vi "Func-엑셀 데이터를 그래프로 출력.vi"() -> ()   [LabVIEW 2015] (continued)
65\t65\t71.845\n65\t65\t71.844\n65\t65\t71.842\n65\t65\t71.84\n65\t65\t71.84\n65\t65\t71.843\n65\t65\t71.838\n65\t65\t71.837\n65\t65\t71.84\n65\t65\t71.846\n65\t65\t71.843\n65\t65\t71.844\n65\t65\t71.846\n65\t65\t71.846\n65\t65\t71.843\n65\t65\t71.832\n65\t65\t71.833\n65\t65\t71.83\n65\t65\t71.829\n65\t65\t71.828\n65\t65\t71.828\n65\t65\t71.832\n65\t65\t71.828\n65\t65\t71.827\n65\t65\t71.823\n65\t65\t71.822\n65\t65\t71.817\n65\t65\t71.814\n65\t65\t71.814\n65\t65\t71.816\n65\t65\t71.817\n65\t65\t71.811\n65\t65\t71.813\n65\t65\t71.814\n65\t65\t71.812\n65\t65\t71.806\n65\t65\t71.799\n65\t65\t71.798\n65\t65\t71.798\n65\t65\t71.793\n65\t65\t71.792\n65\t65\t71.795\n65\t65\t71.796\n65\t65\t71.801\n65\t65\t71.798\n65\t65\t71.797\n65\t65\t71.8\n65\t65\t71.798\n65\t65\t71.799\n65\t65\t71.796\n65\t65\t71.8\n65\t65\t71.803\n65\t65\t71.802\n65\t65\t71.801\n65\t65\t71.797\n65\t65\t71.796\n65\t65\t71.79\n65\t65\t71.786\n65\t65\t71.783\n65\t65\t71.781\n65\t65\t71.782\n65\t65\t71.782\n65\t65\t71.781\n65\t65\t71.781\n65\t65\t71.779\n65\t65\t71.776\n65\t65\t71.777\n65\t65\t71.773\n65\t65\t71.769\n65\t65\t71.769\n65\t65\t71.767\n65\t65\t71.763\n65\t65\t71.761\n65\t65\t71.759\n65\t65\t71.761\n65\t65\t71.754\n65\t65\t71.754\n65\t65\t71.754\n65\t65\t71.751\n65\t65\t71.752\n65\t65\t71.752\n65\t65\t71.755\n65\t65\t71.754\n65\t65\t71.756\n65\t65\t71.754\n65\t65\t71.752\n65\t65\t71.75\n65\t65\t71.75\n65\t65\t71.75\n65\t65\t71.75\n65\t65\t71.749\n65\t65\t71.746\n65\t65\t71.745\n65\t65\t71.741\n65\t65\t71.738\n65\t65\t71.739\n65\t65\t71.742\n65\t65\t71.743\n65\t65\t71.741\n65\t65\t71.741\n65\t65\t71.742\n65\t65\t71.738\n65\t65\t71.738\n65\t65\t71.736\n65\t65\t71.736\n65\t65\t71.733\n65\t65\t71.731\n65\t65\t71.73\n65\t65\t71.725\n65\t65\t71.725\n65\t65\t71.723\n65\t65\t71.721\n65\t65\t71.723\n65\t65\t71.72\n65\t65\t71.72\n65\t65\t71.719\n65\t65\t71.719\n65\t65\t71.716\n65\t65\t71.714\n65\t65\t71.714\n65\t65\t71.714\n65\t65\t71.713\n65\t65\t71.713\n65\t65\t71.714\n65\t65\t71.711\n65\t65\t71.712\n65\t65\t71.711\n65\t65\t71.711\n65\t65\t71.712\n65\t65\t71.712\n65\t65\t71.715\n65\t65\t71.712\n65\t65\t71.709\n65\t65\t71.709\n65\t65\t71.702\n65\t65\t71.7\n65\t65\t71.695\n65\t65\t71.698\n65\t65\t71.698\n65\t65\t71.698\n65\t65\t71.699\n65\t65\t71.698\n65\t65\t71.696\n65\t65\t71.693\n65\t65\t71.691\n65\t65\t71.687\n65\t65\t71.687\n65\t65\t71.687\n65\t65\t71.688\n65\t65\t71.687\n65\t65\t71.689\n65\t65\t71.689\n65\t65\t71.687\n65\t65\t71.686\n65\t65\t71.682\n65\t65\t71.685\n65\t65\t71.683\n65\t65\t71.683\n65\t65\t71.682\n65\t65\t71.679\n65\t65\t71.675\n65\t65\t71.673\n65\t65\t71.669\n65\t65\t71.67\n65\t65\t71.672\n65\t65\t71.677\n65\t65\t71.68\n65\t65\t71.679\n65\t65\t71.679\n65\t65\t71.676\n65\t65\t71.671\n65\t65\t71.671\n65\t65\t71.669\n65\t65\t71.667\n65\t65\t71.666\n65\t65\t71.667\n65\t65\t71.666\n65\t65\t71.666\n65\t65\t71.664\n65\t65\t71.664\n65\t65\t71.66\n65\t65\t71.657\n65\t65\t71.657\n65\t65\t71.652\n65\t65\t71.653\n65\t65\t71.652\n65\t65\t71.656\n65\t65\t71.655\n65\t65\t71.651\n65\t65\t71.652\n65\t65\t71.65\n65\t65\t71.644\n65\t65\t71.643\n65\t65\t71.645\n65\t65\t71.645\n65\t65\t71.645\n65\t65\t71.648\n65\t65\t71.648\n65\t65\t71.645\n65\t65\t71.645\n65\t65\t71.64\n65\t65\t71.637\n65\t65\t71.632\n65\t65\t71.634\n65\t65\t71.633\n65\t65\t71.633\n65\t65\t71.636\n65\t65\t71.637\n65\t65\t71.637\n65\t65\t71.637\n65\t65\t71.637\n65\t65\t71.636\n65\t65\t71.634\n65\t65\t71.633\n65\t65\t71.633\n65\t65\t71.627\n65\t65\t71.623\n65\t65\t71.622\n65\t65\t71.621\n65\t65\t71.617\n65\t65\t71.617\n65\t65\t71.616\n65\t65\t71.618\n65\t65\t71.616\n65\t65\t71.617\n65\t65\t71.621\n65\t65\t71.62\n65\t65\t71.622\n65\t65\t71.621\n65\t65\t71.623\n65\t65\t71.62\n65\t65\t71.613\n65\t65\t71.608\n65\t65\t71.613\n65\t65\t71.613\n65\t65\t71.606\n65\t65\t71.603\n65\t65\t71.602\n65\t65\t71.604\n65\t65\t71.595\n65\t65\t71.595\n65\t65\t71.595\n65\t65\t71.598\n65\t65\t71.597\n65\t65\t71.599\n65\t65\t71.599\n65\t65\t71.595\n65\t65\t71.594\n65\t65\t71.597\n65\t65\t71.601\n65\t65\t71.597\n65\t65\t71.593\n65\t65\t71.593\n65\t65\t71.592\n65\t65\t71.588\n65\t65\t71.584\n65\t65\t71.584\n65\t65\t71.588\n65\t65\t71.586\n65\t65\t71.582\n65\t65\t71.584\n65\t65\t71.583\n65\t65\t71.582\n65\t65\t71.584\n65\t65\t71.585\n65\t65\t71.586\n65\t65\t71.586\n65\t65\t71.584\n65\t65\t71.584\n65\t65\t71.58\n65\t65\t71.58\n65\t65\t71.58\n65\t65\t71.577\n65\t65\t71.574\n65\t65\t71.575\n65\t65\t71.575\n65\t65\t71.57\n65\t65\t71.568\n65\t65\t71.57\n65\t65\t71.57\n65\t65\t71.569\n65\t65\t71.571\n65\t65\t71.572\n65\t65\t71.572\n65\t65\t71.567\n65\t65\t71.568\n65\t65\t71.567\n65\t65\t71.562\n65\t65\t71.561\n65\t65\t71.561\n65\t65\t71.564\n65\t65\t71.562\n65\t65\t71.562\n65\t65\t71.56\n65\t65\t71.557\n65\t65\t71.557\n65\t65\t71.553\n65\t65\t71.554\n65\t65\t71.549\n65\t65\t71.548\n65\t65\t71.548\n65\t65\t71.548\n65\t65\t71.551\n65\t65\t71.553\n65\t65\t71.551\n65\t65\t71.554\n65\t65\t71.556\n65\t65\t71.555\n65\t65\t71.552\n65\t65\t71.553\n65\t65\t71.556\n65\t65\t71.555\n65\t65\t71.55\n65\t65\t71.546\n65\t65\t71.542\n65\t65\t71.536\n65\t65\t71.535\n65\t65\t71.532\n65\t65\t71.533\n65\t65\t71.532\n65\t65\t71.536\n65\t65\t71.539\n65\t65\t71.536\n65\t65\t71.534\n65\t65\t71.534\n65\t65\t71.536\n65\t65\t71.534\n65\t65\t71.531\n65\t65\t71.534\n65\t65\t71.537\n65\t65\t71.536\n65\t65\t71.537\n65\t65\t71.536\n65\t65\t71.535\n65\t65\t71.531\n65\t65\t71.528\n65\t65\t71.528\n65\t65\t71.526\n65\t65\t71.528\n65\t65\t71.527\n65\t65\t71.529\n65\t65\t71.528\n65\t65\t71.528\n65\t65\t71.523\n65\t65\t71.518\n65\t65\t71.518\n65\t65\t71.519\n65\t65\t71.52\n65\t65\t71.519\n65\t65\t71.522\n65\t65\t71.527\n65\t65\t71.523\n65\t65\t71.52\n65\t65\t71.517\n65\t65\t71.517\n65\t65\t71.512\n65\t65\t71.511\n65\t65\t71.511\n65\t65\t71.508\n65\t65\t71.509\n65\t65\t71.507\n65\t65\t71.509\n65\t65\t71.507\n65\t65\t71.509\n65\t65\t71.511\n65\t65\t71.506\n65\t65\t71.507\n65\t65\t71.505\n65\t65\t71.504\n65\t65\t71.5\n65\t65\t71.5\n65\t65\t71.502\n65\t65\t71.499\n65\t65\t71.499\n65\t65\t71.495\n65\t65\t71.495\n65\t65\t71.491\n65\t65\t71.489\n65\t65\t71.491\n65\t65\t71.49\n65\t65\t71.491\n65\t65\t71.491\n65\t65\t71.492\n65\t65\t71.493\n65\t65\t71.491\n65\t65\t71.488\n65\t65\t71.492\n65\t65\t71.491\n65\t65\t71.49\n65\t65\t71.489\n65\t65\t71.486\n65\t65\t71.486\n65\t65\t71.48\n65\t65\t71.476\n65\t65\t71.476\n65\t65\t71.473\n65\t65\t71.474\n65\t65\t71.475\n65\t65\t71.477\n65\t65\t71.476\n65\t65\t71.473\n65\t65\t71.471\n65\t65\t71.47\n65\t65\t71.468\n65\t65\t71.47\n65\t65\t71.471\n65\t65\t71.474\n65\t65\t71.473\n65\t65\t71.473\n65\t65\t71.471\n65\t65\t71.467\n65\t65\t71.465\n65\t65\t71.463\n65\t65\t71.465\n65\t65\t71.466\n65\t65\t71.468\n65\t65\t71.469\n65\t65\t71.468\n65\t65\t71.464\n65\t65\t71.459\n65\t65\t71.458\n65\t65\t71.454\n65\t65\t71.45\n65\t65\t71.452\n65\t65\t71.453\n65\t65\t71.456\n65\t65\t71.457\n65\t65\t71.464\n65\t65\t71.462\n65\t65\t71.457\n65\t65\t71.457\n65\t65\t71.455\n65\t65\t71.455\n65\t65\t71.457\n65\t65\t71.454\n65\t65\t71.456\n65\t65\t71.461\n65\t65\t71.457\n65\t65\t71.452\n65\t65\t71.446\n65\t65\t71.447\n65\t65\t71.447\n65\t65\t71.443\n65\t65\t71.445\n65\t65\t71.446\n65\t65\t71.446\n65\t65\t71.443\n65\t65\t71.438\n65\t65\t71.441\n65\t65\t71.438\n65\t65\t71.437\n65\t65\t71.434\n65\t65\t71.436\n65\t65\t71.441\n65\t65\t71.437\n65\t65\t71.436\n65\t65\t71.437\n65\t65\t71.441\n65\t65\t71.442\n65\t65\t71.439\n65\t65\t71.441\n65\t65\t71.443\n65\t65\t71.443\n65\t65\t71.438\n65\t65\t71.44\n65\t65\t71.44\n65\t65\t71.439\n65\t65\t71.439\n65\t65\t71.437\n65\t65\t71.436\n65\t65\t71.433\n65\t65\t71.43\n65\t65\t71.43\n65\t65\t71.426\n65\t65\t71.424\n65\t65\t71.425\n65\t65\t71.422\n65\t65\t71.424\n65\t65\t71.422\n65\t65\t71.428\n65\t65\t71.429\n65\t65\t71.427\n65\t65\t71.426\n65\t65\t71.423\n65\t65\t71.42\n65\t65\t71.412\n65\t65\t71.409\n65\t65\t71.409\n65\t65\t71.405\n65\t65\t71.407\n65\t65\t71.409\n65\t65\t71.409\n65\t65\t71.407\n65\t65\t71.413\n65\t65\t71.415\n65\t65\t71.416\n65\t65\t71.417\n65\t65\t71.415\n65\t65\t71.417\n65\t65\t71.409\n65\t65\t71.409\n65\t65\t71.403\n65\t65\t71.398\n65\t65\t71.4\n65\t65\t71.404\n65\t65\t71.407\n65\t65\t71.405\n65\t65\t71.407\n65\t65\t71.407\n65\t65\t71.405\n65\t65\t71.405\n65\t65\t71.401\n65\t65\t71.402\n65\t65\t71.402\n65\t65\t71.4\n65\t65\t71.402\n65\t65\t71.398\n65\t65\t71.398\n65\t65\t71.398\n65\t65\t71.398\n65\t65\t71.4\n65\t65\t71.396\n65\t65\t71.391\n65\t65\t71.394\n65\t65\t71.396\n65\t65\t71.39\n65\t65\t71.391\n65\t65\t71.393\n65\t65\t71.396\n65\t65\t71.393\n65\t65\t71.387\n65\t65\t71.39\n65\t65\t71.388\n65\t65\t71.386\n65\t65\t71.383\n65\t65\t71.38\n65\t65\t71.38\n65\t65\t71.38\n65\t65\t71.38\n65\t65\t71.38\n65\t65\t71.381\n65\t65\t71.385\n65\t65\t71.387\n65\t65\t71.387\n65\t65\t71.385\n65\t65\t71.387\n65\t65\t71.384\n65\t65\t71.385\n65\t65\t71.385\n65\t65\t71.383\n65\t65\t71.382\n65\t65\t71.379\n65\t65\t71.38\n65\t65\t71.377\n65\t65\t71.375\n65\t65\t71.378\n65\t65\t71.38\n65\t65\t71.379\n65\t65\t71.376\n65\t65\t71.373\n65\t65\t71.372\n65\t65\t71.367\n65\t65\t71.366\n65\t65\t71.363\n65\t65\t71.364\n65\t65\t71.365\n65\t65\t71.366\n65\t65\t71.367\n65\t65\t71.369\n65\t65\t71.368\n65\t65\t71.368\n65\t65\t71.37\n65\t65\t71.366\n65\t65\t71.364\n65\t65\t71.359\n65\t65\t71.362\n65\t65\t71.357\n65\t65\t71.356\n65\t65\t71.356\n65\t65\t71.355\n65\t65\t71.357\n65\t65\t71.356\n65\t65\t71.363\n65\t65\t71.364\n65\t65\t71.364\n65\t65\t71.364\n65\t65\t71.364\n65\t65\t71.36\n65\t65\t71.359\n65\t65\t71.355\n65\t65\t71.359\n65\t65\t71.353\n65\t65\t71.35\n65\t65\t71.356\n65\t65\t71.354\n65\t65\t71.358\n65\t65\t71.351\n65\t65\t71.353\n65\t65\t71.353\n65\t65\t71.35\n65\t65\t71.347\n65\t65\t71.341\n65\t65\t71.345\n65\t65\t71.345\n65\t65\t71.346\n65\t65\t71.342\n65\t65\t71.342\n65\t65\t71.343\n65\t65\t71.341\n65\t65\t71.341\n65\t65\t71.34\n65\t65\t71.342\n65\t65\t71.342\n65\t65\t71.341\n65\t65\t71.342\n65\t65\t71.344\n65\t65\t71.343\n65\t65\t71.343\n64.917\t64.93\t70.994\n64.833\t64.95\t70.988\n64.75\t64.99\t71\n64.667\t64.94\t70.985\n64.583\t64.85\t70.985\n64.5\t64.74\t70.993\n64.417\t64.6\t70.981\n64.333\t64.45\t70.977\n64.25\t64.28\t70.982\n64.167\t64.11\t70.976\n64.083\t63.94\t70.983\n64\t63.75\t70.967\n63.917\t63.55\t70.968\n63.833\t63.35\t70.964\n63.75\t63.17\t70.967\n63.667\t62.98\t70.955\n63.583\t62.82\t70.955\n63.5\t62.66\t70.948\n63.417\t62.52\t70.946\n63.333\t62.38\t70.934\n63.25\t62.26\t70.937\n63.167\t62.16\t70.923\n63.083\t62.06\t70.918\n63\t61.98\t70.91\n62.917\t61.9\t70.896\n62.833\t61.82\t70.882\n62.75\t61.75\t70.875\n62.667\t61.69\t70.86\n62.583\t61.62\t70.85\n62.5\t61.56\t70.836\n62.417\t61.51\t70.822\n62.333\t61.46\t70.809\n62.25\t61.41\t70.791\n62.167\t61.35\t70.771\n62.083\t61.3\t70.764\n62\t61.24\t70.734\n61.917\t61.18\t70.716\n61.833\t61.11\t70.704\n61.75\t61.04\t70.682\n61.667\t60.96\t70.661\n61.583\t60.88\t70.638\n61.5\t60.81\t70.618\n61.417\t60.75\t70.586\n61.333\t60.65\t70.568\n61.25\t60.57\t70.541\n61.167\t60.48\t70.516\n61.083\t60.4\t70.499\n61\t60.3\t70.469\n60.917\t60.21\t70.444\n60.833\t60.14\t70.418\n60.75\t60.05\t70.392\n60.667\t59.95\t70.367\n60.583\t59.87\t70.33\n60.5\t59.78\t70.298\n60.417\t59.7\t70.273\n60.333\t59.62\t70.252\n60.25\t59.53\t70.217\n60.167\t59.45\t70.191\n60.083\t59.36\t70.163\n60\t59.27\t70.119\n59.917\t59.19\t70.095\n59.833\t59.1\t70.055\n59.75\t59.02\t70.024\n59.667\t58.95\t69.993\n59.583\t58.86\t69.957\n59.5\t58.78\t69.915\n59.417\t58.71\t69.886\n59.333\t58.63\t69.849\n59.25\t58.55\t69.816\n59.167\t58.46\t69.777\n59.083\t58.37\t69.74\n59\t58.29\t69.689\n58.917\t58.21\t69.654\n58.833\t58.14\t69.623\n58.75\t58.05\t69.577\n58.667\t57.98\t69.545\n58.583\t57.9\t69.5\n58.5\t57.84\t69.464\n58.417\t57.75\t69.424\n58.333\t57.66\t69.378\n58.25\t57.57\t69.335\n58.167\t57.5\t69.28\n58.083\t57.41\t69.25\n58\t57.34\t69.204\n57.917\t57.26\t69.165\n57.833\t57.17\t69.124\n57.75\t57.09\t69.081\n57.667\t57.02\t69.033\n57.583\t56.93\t68.982\n57.5\t56.86\t68.937\n57.417\t56.77\t68.895\n57.333\t56.67\t68.846\n57.25\t56.59\t68.795\n57.167\t56.5\t68.747\n57.083\t56.42\t68.713\n57\t56.34\t68.652\n56.917\t56.26\t68.604\n56.833\t56.17\t68.555\n56.75\t56.09\t68.512\n56.667\t56.01\t68.463\n56.583\t55.95\t68.409\n56.5\t55.87\t68.359\n56.417\t55.79\t68.312\n56.333\t55.71\t68.257\n56.25\t55.63\t68.221\n56.167\t55.56\t68.155\n56.083\t55.47\t68.114\n56\t55.38\t68.054\n55.917\t55.28\t68.01\n55.833\t55.2\t67.953\n55.75\t55.11\t67.896\n55.667\t55.03\t67.848\n55.583\t54.95\t67.797\n55.5\t54.86\t67.739\n55.417\t54.79\t67.679\n55.333\t54.71\t67.63\n55.25\t54.63\t67.577\n55.167\t54.55\t67.522\n55.083\t54.47\t67.467\n55\t54.39\t67.412\n54.917\t54.3\t67.352\n54.833\t54.21\t67.297\n54.75\t54.13\t67.246\n54.667\t54.05\t67.191\n54.583\t53.96\t67.125\n54.5\t53.88\t67.075\n54.417\t53.8\t67.01\n54.333\t53.71\t66.959\n54.25\t53.63\t66.9\n54.167\t53.55\t66.84\n54.083\t53.47\t66.792\n54\t53.39\t66.712\n53.917\t53.32\t66.659\n53.833\t53.22\t66.604\n53.75\t53.14\t66.549\n53.667\t53.06\t66.483\n53.583\t52.99\t66.425\n53.5\t52.91\t66.371\n53.417\t52.83\t66.307\n53.333\t52.74\t66.25\n53.25\t52.65\t66.189\n53.167\t52.57\t66.131\n53.083\t52.5\t66.065\n53\t52.42\t66.004\n52.917\t52.34\t65.94\n52.833\t52.26\t65.88\n52.75\t52.17\t65.821\n52.667\t52.09\t65.754\n52.583\t52.01\t65.684\n52.5\t51.93\t65.636\n52.417\t51.85\t65.568\n52.333\t51.76\t65.503\n52.25\t51.68\t65.447\n52.167\t51.6\t65.382\n52.083\t51.52\t65.316\n52\t51.43\t65.261\n51.917\t51.35\t65.191\n51.833\t51.27\t65.127\n51.75\t51.18\t65.059\n51.667\t51.1\t65.005\n51.583\t51.01\t64.942\n51.5\t50.93\t64.863\n51.417\t50.85\t64.805\n51.333\t50.76\t64.738\n51.25\t50.69\t64.68\n51.167\t50.6\t64.604\n51.083\t50.52\t64.546\n51\t50.44\t64.483\n50.917\t50.36\t64.409\n50.833\t50.28\t64.348\n50.75\t50.21\t64.279\n50.667\t50.13\t64.218\n50.583\t50.04\t64.142\n50.5\t49.96\t64.077\n50.417\t49.88\t64.018\n50.333\t49.8\t63.946\n50.25\t49.72\t63.884\n50.167\t49.62\t63.813\n50.083\t49.54\t63.753\n50\t49.45\t0\n49.917\t49.37\t63.585\n49.833\t49.28\t0\n49.75\t49.21\t63.387\n49.667\t49.13\t63.307\n49.583\t49.04\t63.24\n49.5\t48.95\t63.189\n49.417\t48.88\t63.148\n49.333\t48.79\t63.102\n49.25\t48.72\t63.054\n49.167\t48.64\t63.008\n49.083\t48.56\t62.953\n49\t48.47\t62.905\n48.917\t48.39\t62.852\n48.833\t48.31\t62.786\n48.75\t48.23\t62.732\n48.667\t48.16\t62.667\n48.583\t48.08\t62.604\n48.5\t48\t62.556\n48.417\t47.92\t62.491\n48.333\t47.85\t62.414\n48.25\t47.76\t62.358\n48.167\t47.68\t62.294\n48.083\t47.6\t62.227\n48\t47.5\t62.154\n47.917\t47.42\t62.093\n47.833\t47.33\t62.027\n47.75\t47.24\t61.945\n47.667\t47.16\t61.881\n47.583\t47.08\t61.818\n47.5\t47\t61.742\n47.417\t46.92\t61.674\n47.333\t46.83\t61.601\n47.25\t46.74\t61.525\n47.167\t46.66\t61.452\n47.083\t46.58\t61.376\n47\t46.51\t61.31\n46.917\t46.43\t61.228\n46.833\t46.35\t61.168\n46.75\t46.28\t61.094\n46.667\t46.2\t61.021\n46.583\t46.13\t60.939\n46.5\t46.04\t60.878\n46.417\t45.97\t60.806\n46.333\t45.88\t60.729\n46.25\t45.81\t60.654\n46.167\t45.73\t60.581\n46.083\t45.66\t60.504\n46\t45.57\t60.426\n45.917\t45.5\t60.362\n45.833\t45.42\t60.289\n45.75\t45.34\t60.216\n45.667\t45.27\t60.142\n45.583\t45.19\t60.065\n45.5\t45.1\t59.984\n45.417\t45.01\t59.914\n45.333\t44.91\t59.838\n45.25\t44.82\t59.765\n45.167\t44.73\t59.682\n45.083\t44.65\t59.616\n45\t44.56\t59.532\n45\t44.48\t59.473\n45\t44.48\t59.467\n45\t44.47\t59.462\n45\t44.46\t59.455\n45\t44.45\t59.443\n45\t44.45\t59.436\n45\t44.44\t59.427\n45\t44.43\t59.418\n45\t44.42\t59.41\n45\t44.41\t59.401\n45\t44.4\t59.396\n45\t44.39\t59.392\n45\t44.38\t59.382\n45\t44.37\t59.379\n45\t44.36\t59.373\n45\t44.35\t59.364\n45\t44.35\t59.357\n45\t44.35\t59.348\n45\t44.34\t59.34\n45\t44.33\t59.329\n45\t44.32\t59.322\n45\t44.31\t59.318\n45\t44.3\t59.31\n45\t44.29\t59.304\n45\t44.29\t59.293\n45\t44.28\t59.288\n45\t44.27\t59.28\n45\t44.26\t59.269\n45\t44.26\t59.261\n45\t44.25\t59.257\n45\t44.24\t59.249\n45\t44.24\t59.24\n45\t44.23\t59.235\n45\t44.22\t59.231\n45\t44.21\t59.225\n45\t44.21\t59.217\n45\t44.2\t59.209\n45\t44.19\t59.204\n45\t44.19\t59.193\n45\t44.18\t59.182\n45\t44.18\t59.178\n45\t44.17\t59.166\n45\t44.16\t59.156\n45\t44.16\t59.151\n45\t44.16\t59.141\n45\t44.15\t59.133\n45\t44.15\t59.127\n45\t44.14\t59.121\n45\t44.14\t59.12\n45\t44.13\t59.113\n45\t44.13\t59.105\n45\t44.12\t59.1\n45\t44.12\t59.084\n45\t44.12\t59.079\n45\t44.11\t59.068\n45\t44.11\t59.057\n45\t44.11\t59.05\n45\t44.1\t59.044\n45\t44.1\t59.039\n45\t44.1\t59.03\n45\t44.09\t59.025\n45\t44.09\t59.016\n45\t44.08\t59.009\n45\t44.08\t59.003\n45\t44.08\t58.995\n45\t44.08\t58.99\n45\t44.08\t58.986\n45\t44.08\t58.978\n45\t44.08\t58.97\n45\t44.07\t58.961\n45\t44.07\t58.954\n45\t44.07\t58.945\n45\t44.07\t58.931\n45\t44.07\t58.925\n45\t44.07\t58.919\n45\t44.07\t58.909\n45\t44.07\t58.904\n45\t44.07\t58.9\n45\t44.07\t58.892\n45\t44.07\t58.883\n45\t44.07\t58.876\n45\t44.07\t58.867\n45\t44.07\t58.857\n45\t44.07\t58.849\n45\t44.07\t58.846\n45\t44.07\t58.838\n45\t44.07\t58.829\n45\t44.07\t58.823\n45\t44.07\t58.82\n45\t44.07\t58.808\n45\t44.07\t58.799\n45\t44.07\t58.791\n45\t44.07\t58.782\n45\t44.07\t58.775\n45\t44.07\t58.763\n45\t44.07\t58.755\n45\t44.07\t58.746\n45\t44.07\t58.743\n45\t44.07\t58.735\n45\t44.07\t58.729\n45\t44.07\t58.723\n45\t44.07\t58.719\n45\t44.07\t58.714\n45\t44.07\t58.704\n45\t44.08\t58.698\n45\t44.07\t58.687\n45\t44.08\t58.684\n45\t44.08\t58.671\n45\t44.08\t58.667\n45\t44.08\t58.659\n45\t44.08\t58.65\n45\t44.09\t58.648\n45\t44.09\t58.634\n45\t44.09\t58.633\n45\t44.09\t58.62\n45\t44.09\t58.611\n45\t44.1\t58.608\n45\t44.1\t58.597\n45\t44.1\t58.585\n45\t44.11\t58.579\n45\t44.11\t58.574\n45\t44.11\t58.565\n45\t44.11\t58.554\n45\t44.12\t58.548\n45\t44.12\t58.542\n45\t44.12\t58.534\n45\t44.13\t58.529\n45\t44.13\t58.524\n45\t44.13\t58.519\n45\t44.14\t58.509\n45\t44.14\t58.502\n45\t44.14\t58.496\n45\t44.15\t58.485\n45\t44.15\t58.475\n45\t44.16\t58.468\n45\t44.16\t58.461\n45\t44.16\t58.455\n45\t44.16\t58.447\n45\t44.16\t58.438\n45\t44.16\t58.434\n45\t44.16\t58.431\n45\t44.17\t58.426\n45\t44.18\t58.418\n45\t44.18\t58.413\n45\t44.19\t58.405\n45\t44.19\t58.396\n45\t44.19\t58.386\n45\t44.19\t58.377\n45\t44.19\t58.37\n45\t44.2\t58.36\n45\t44.2\t58.352\n45\t44.21\t58.348\n45\t44.21\t58.342\n45\t44.21\t58.332\n45\t44.22\t58.323\n45\t44.22\t58.317\n45\t44.22\t58.309\n45\t44.23\t58.3\n45\t44.23\t58.284\n45\t44.23\t58.281\n45\t44.24\t58.278\n45\t44.24\t58.268\n45\t44.25\t58.263\n45\t44.25\t58.259\n45\t44.25\t58.253\n45\t44.26\t58.245\n45\t44.26\t58.237\n45\t44.26\t58.228\n45\t44.26\t58.226\n45\t44.26\t58.216\n45\t44.26\t58.205\n45\t44.26\t58.198\n45\t44.26\t58.193\n45\t44.27\t58.184\n45\t44.27\t58.178\n45\t44.27\t58.171\n45\t44.28\t58.163\n45\t44.28\t58.155\n45\t44.29\t58.144\n45\t44.29\t58.138\n45\t44.29\t58.128\n45\t44.29\t58.12\n45\t44.3\t58.113\n45\t44.3\t58.105\n45\t44.3\t58.098\n45\t44.31\t58.092\n45\t44.31\t58.084\n45\t44.32\t58.073\n45\t44.32\t58.067\n45\t44.33\t58.06\n45\t44.33\t58.051\n45\t44.34\t58.045\n45\t44.34\t58.04\n45\t44.34\t58.034\n45\t44.35\t58.031\n45\t44.35\t58.026\n45\t44.35\t58.02\n45\t44.35\t58.013\n45\t44.35\t57.999\n45\t44.35\t57.993\n45\t44.35\t57.986\n45\t44.36\t57.974\n45\t44.36\t57.971\n45\t44.37\t57.963\n45\t44.37\t57.955\n45\t44.38\t57.948\n45\t44.38\t57.939\n45\t44.38\t57.93\n45\t44.38\t57.921\n45\t44.39\t57.917\n45\t44.39\t57.911\n45\t44.39\t57.904\n45\t44.4\t57.897\n45\t44.4\t57.892\n45\t44.41\t57.887\n45\t44.41\t57.88\n45\t44.41\t57.871\n45\t44.42\t57.867\n45\t44.42\t57.864\n45\t44.42\t57.854\n45\t44.43\t57.845\n45\t44.43\t57.838\n45\t44.43\t57.829\n45\t44.44\t57.823\n45\t44.44\t57.813\n45\t44.44\t57.808\n45\t44.45\t57.802\n45\t44.45\t57.796\n45\t44.45\t57.787\n45\t44.45\t57.776\n45\t44.45\t57.771\n45\t44.46\t57.761\n45\t44.46\t57.76\n45\t44.47\t57.748\n45\t44.47\t57.744\n45\t44.47\t57.739\n45\t44.48\t57.728\n45\t44.48\t57.723\n45\t44.48\t57.71\n45\t44.49\t57.701\n45\t44.49\t57.696\n45\t44.49\t57.692\n45\t44.5\t57.682\n45\t44.5\t57.674\n45\t44.5\t57.67\n45\t44.51\t57.666\n45\t44.51\t57.661\n45\t44.51\t57.653\n45\t44.52\t57.643\n45\t44.52\t57.637\n45\t44.53\t57.632\n45\t44.53\t57.624\n45\t44.53\t57.614\n45\t44.54\t57.608\n45\t44.54\t57.601\n45\t44.54\t57.594\n45\t44.54\t57.584\n45\t44.55\t57.579\n45\t44.55\t57.573\n45\t44.55\t
